vi "Normalized Case Decode.vi"(0 "m":u32[](array[numeric]), 1 "n-m":u32[](array[numeric]), 2 "table":dbl[][](array[numeric]) format="%.2f") -> (3 "m*":u32[](array[numeric]), 4 "n-m*":u32[](array[numeric]), 5 "table*":dbl[][](array[numeric]) format="%.2f", 6 "error":i32)   [LabVIEW 2014, in "NI_Gmath.lvlib"]
uses:
  NI_Gmath.lvlib
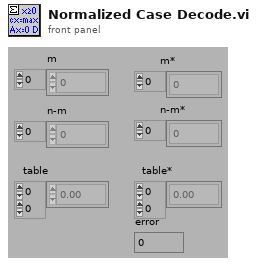
[diagram p1: front panel]
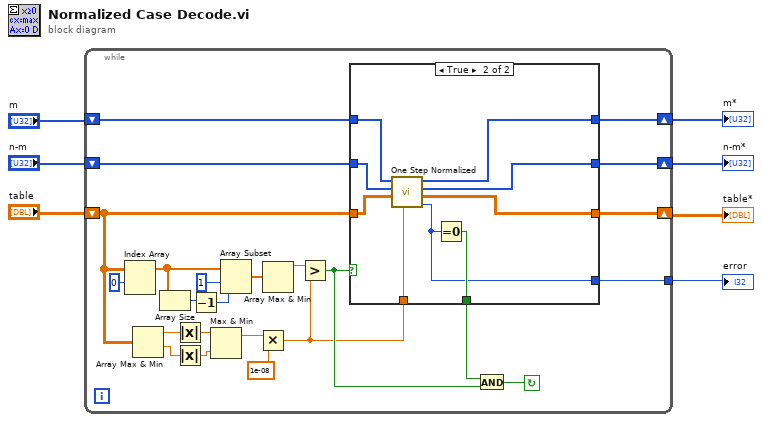
[diagram p0: block diagram]
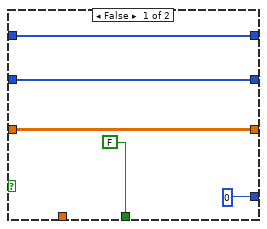
[diagram p2: hidden frame]
diagram:
  n1 = while {
    tunnel: [w17] -> w4
    shift-left: "table" -> [w14]
    shift-right: [w18] -> w1
    shift-left: "n-m" -> [w23]
    shift-right: [w22] -> w2
    shift-left: "m" -> [w25]
    shift-right: [w24] -> w3
    stop <- w19 continue-if-true
    n2 = Index Array(array=w14, index (row)=0) -> (element=w29:dbl[])  [unwired: 1 in]
    n3 = Array Max & Min(array=w14) -> (max value=w13:dbl, min value=w12:dbl)  [unwired: 2 out]
    n4 = Array Size(array=w29) -> (size(s)=w28:i32)
    n5 = Absolute Value(x=w13) -> (abs(x)=w11:dbl)
    n6 = Absolute Value(x=w12) -> (abs(x)=w10:dbl)
    n7 = Decrement(x=w28) -> (x-1=w27:i32)
    n8 = Max & Min(x=w11, y=w10) -> (max(x,y)=w9:dbl)  [unwired: 1 out]
    n9 = Array Subset(array=w29, index=1, length=w27) -> (w26:dbl[])
    n10 = Multiply(x=w9, y=1e-08) -> (x*y=w8:dbl)
    n11 = Array Max & Min(array=w26) -> (max value=w16:dbl)  [unwired: 3 out]
    n12 = Greater?(x=w16, y=w8) -> (0:w20:bool)
    n13 = case shown="True" w20 {
      tunnel: w25 -> [w36 w45]
      tunnel: [w36 w39] -> w24
      tunnel: w14 -> [w35 w42]
      tunnel: [w35 w37] -> w18
      tunnel: w23 -> [w34 w44]
      tunnel: [w34 w38] -> w22
      tunnel: [FALSE w43] -> w21
      tunnel: [0 w41] -> w17
      tunnel: w8 -> [_ w40]
      frame False {
      }
      frame True {
        n14 = call "One Step Normalized.vi"("eps"=w40, "table"=w42, "n-m"=w44, "m"=w45) -> ("error"=w41:i32, "table*"=w37:dbl[][], "n-m*"=w38:u32[], "m*"=w39:u32[])  [unwired: 4 in]
        n15 = Equal To 0?(x=w41) -> (x = 0?=w43:bool)
      }
    }
    n16 = And(x=w21, y=w20) -> (x .and. y?=w19:bool)
  }
  "n-m*" <- w2
  "m*" <- w3
  "error" <- w4
  "table*" <- w1
